vi "Read logs.vi"(8 "error in (no error)":errorcluster, 11 "Logger in":refnum<class "Logger.lvclass">) -> (0 "error out":errorcluster, 2 "logs":string[](array[string]), 3 "Logger out":refnum<class "Logger.lvclass">)   [LabVIEW 2017, in "Logger.lvclass"]
uses:
  Logger.lvclass
  Logger.lvclass/Logger.ctl
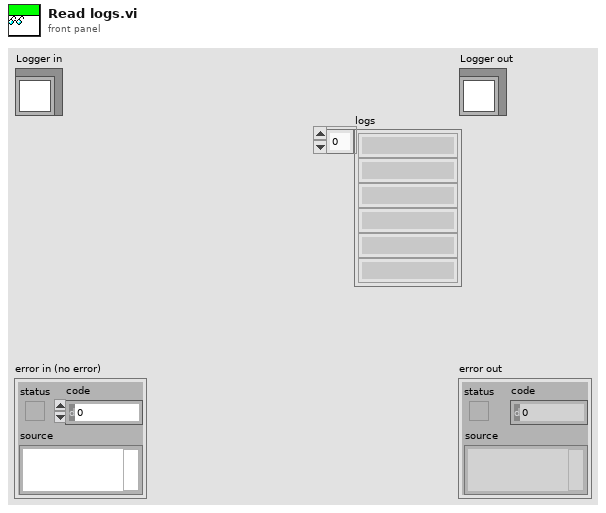
[diagram p1: front panel]
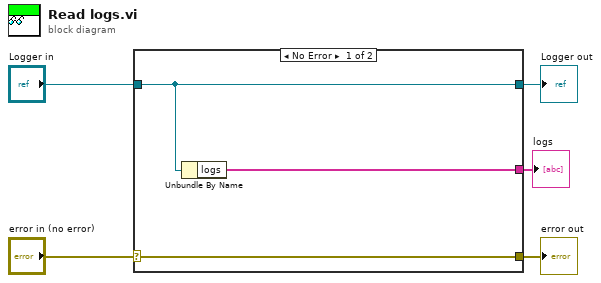
[diagram p0: block diagram]
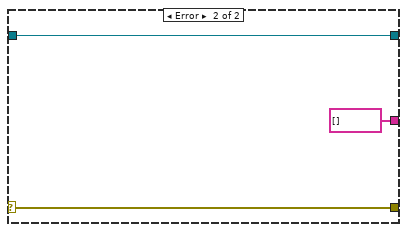
[diagram p2: hidden frame]
diagram:
  n1 = case shown="No Error" "error in (no error)" {
    selector: "error in (no error)" -> [w8 w10]
    tunnel: [w8 w10] -> w4
    tunnel: [w7 w11] -> w2
    tunnel: "Logger in" -> [w7 w11]
    tunnel: [w6 string[] [] ("logs")] -> w1
    frame No Error {
      n2 = Unbundle By Name(w7) -> ("logs"=w6:string[])
    }
    frame Error {
    }
  }
  "error out" <- w4
  "Logger out" <- w2
  "logs" <- w1
